vi "Set Transform.vi"(8 "error in (no error)":errorcluster, 10 "Real Matrix 2x3":T1, 11 "Drawer .Net in":refnum<class "Drawer .Net.lvclass">) -> (0 "error out":errorcluster, 3 "Drawer .Net out":refnum<class "Drawer .Net.lvclass">)   [LabVIEW 2023, in "Glyph .NET Drawer.lvlib" / "Drawer .Net.lvclass"]
uses:
  Drawer .Net.lvclass
  <vilib>/Analysis/Matrix/Datatypes/RealMatrix.ctl
  Drawer .Net.lvclass/Drawer .Net.ctl
  System.Drawing
  <vilib>/Analysis/Matrix/NI_Matrix.lvlib
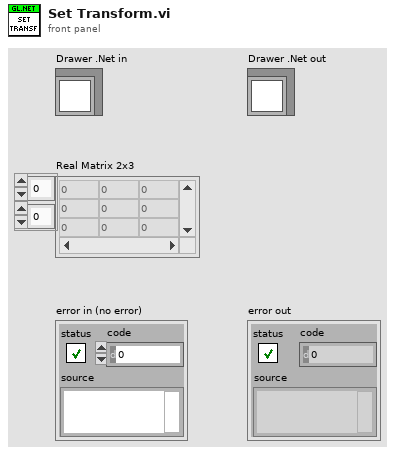
[diagram p1: front panel]
types:
  T1 = typedef "NI_Matrix.lvlib/RealMatrix.ctl" = dbl[][]
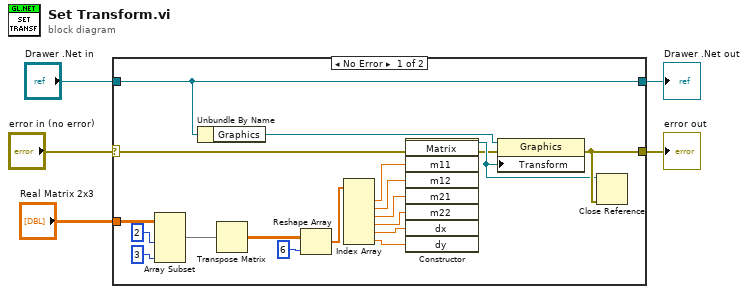
[diagram p0: block diagram]
diagram:
  n1 = case shown="No Error" "error in (no error)" {
    selector: "error in (no error)" -> [w22 w26]
    tunnel: [w21 w26] -> w4
    tunnel: [w24 w25] -> w2
    tunnel: "Drawer .Net in" -> [w24 w25]
    tunnel: "Real Matrix 2x3" -> [w18 _]
    frame No Error {
      n2 = Array Subset(array=w18, length (row)=2 ("length"), length (col)=3 ("length")) -> (w15:T1)  [unwired: 2 in]
      n3 = Unbundle By Name(w24) -> ("Graphics"=w23:refnum<k24>)
      n4 = Transpose Matrix(1:w15) -> (0:w12:T1)
      n5 = Reshape Array(w12, 6 ("dimension size")) -> (w13:dbl[])
      n6 = Index Array(array=w13) -> (element #1=w9:dbl, element #2=w8:dbl, element #3=w7:dbl, element #4=w6:dbl, element #5=w11:dbl, element #6=w10:dbl)  [unwired: 6 in]
      n7 = constructor class="Matrix"(error in=w22, "m11"=w9, "m12"=w8, "m21"=w7, "m22"=w6, "dx"=w11, "dy"=w10) -> (reference out=w20:refnum<k24>, error out=w19:errorcluster)  [unwired: 2 in, 7 out]
      n8 = property class="Graphics"(reference=w23, error in=w19, "Transform"=w20) -> (error out=w21:errorcluster)  [unwired: 1 out]
      n9 = Close Reference(reference=w20, error in (no error)=w21) -> ()  [unwired: 1 out]
    }
    frame Error {
    }
  }
  "error out" <- w4
  "Drawer .Net out" <- w2
